vi "Schedule size.vi"(8 "error in (no error)":errorcluster, 11 "Schedule in":refnum<class "Schedule.lvclass">) -> (0 "error out":errorcluster, 2 "Size":i32, 3 "Schedule out":refnum<class "Schedule.lvclass">)   [LabVIEW 2020, in "CIRCUS_uServices.lvlib" / "Run Utilities.lvlib" / "Schedule.lvclass"]
doc: "Get number of cells in the schedule"
uses:
  Schedule.lvclass
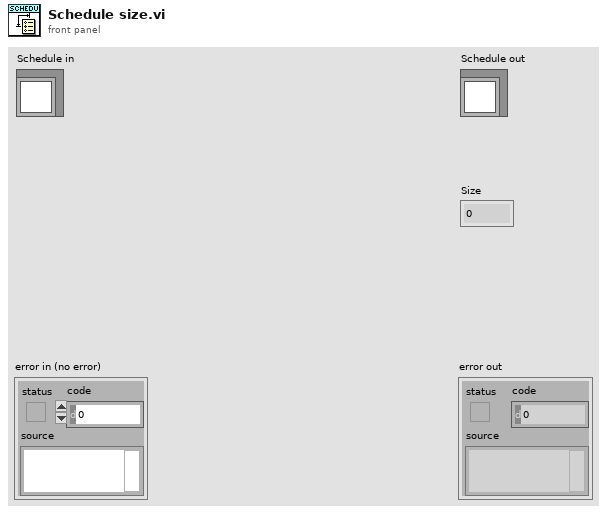
[diagram p1: front panel]
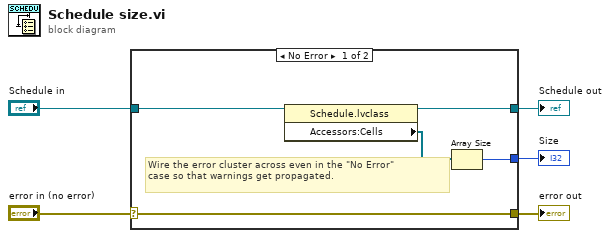
[diagram p0: block diagram]
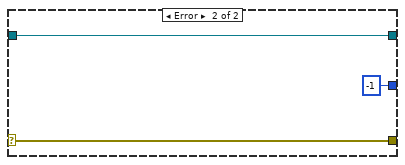
[diagram p2: hidden frame]
diagram:
  n1 = case shown="No Error" "error in (no error)" {
    selector: "error in (no error)" -> [w9 w13]
    tunnel: [w9 w13] -> w4
    tunnel: [w8 w12] -> w2
    tunnel: "Schedule in" -> [w10 w12]
    tunnel: [w7 -1] -> w1
    frame No Error {
      # "Wire the error cluster across even in the \"No Error\"\ncase so that warnings get propagated."
      n2 = property class="Schedule.lvclass"(reference=w10) -> (reference out=w8:refnum<class "Schedule.lvclass">, "Accessors:Cells"=w6:refnum<class "Schedule Cell.lvclass">[])  [unwired: 1 in, 1 out]
      n3 = Array Size(array=w6) -> (size(s)=w7:i32)
    }
    frame Error {
    }
  }
  "error out" <- w4
  "Schedule out" <- w2
  "Size" <- w1
